vi "VI Tree.vi"   [LabVIEW 2014, in "KIT QV.lvlib"]
doc: "This is the instrument driver for the <INSTRUMENT NAME>. The VI Tree displays all the user-callable VIs of the instrument driver in an organized table."
uses:
  KIT QV.lvlib
panel:
  # "(c) 2015 GSI Helmholtzzentrum für Schwerionenforschung GmbH.  ALL RIGHTS RESERVED."
  # "SEE DIAGRAM\nFOR VI TREE."
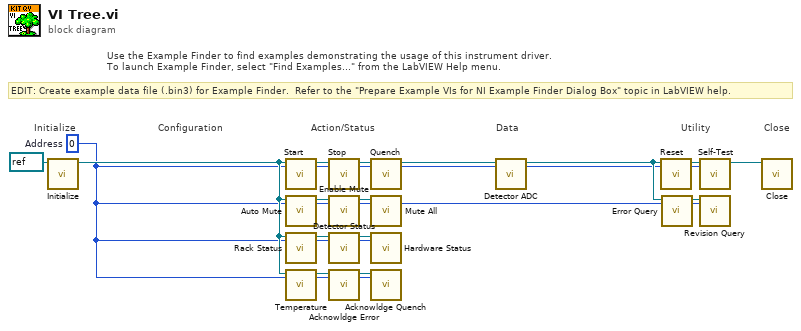
[diagram p0: block diagram]
diagram:
  w1 = u16 0  # Address
  # "EDIT: Create example data file (.bin3) for Example Finder.  Refer to the \"Prepare Example VIs for NI Example Finder Dialog Box\" topic in LabVIEW help."
  # "Use the Example Finder to find examples demonstrating the usage of this instrument driver.\nTo launch Example Finder, select \"Find Examples...\" from the LabVIEW Help menu."
  # "Configuration"
  # "Utility"
  # "Data"
  # "Action/Status"
  # "Close"
  # "Initialize"
  n1 = call "Initialize.vi"("VISA Resource Name"=refnum<visa-resource-name> refnum ("VISA resource name")) -> ("VISA Resource out"=w6:refnum<visa-resource-name>)  [unwired: 9 in, 1 out]
  n2 = call "Start.vi"("Address"=w1, "VISA Resource in"=w6) -> ("VISA Resource out"=w11:refnum<visa-resource-name>)  [unwired: 8 in, 1 out]
  n3 = call "Auto Mute.vi"("Address"=w1, "VISA Resource in"=w6) -> ("VISA Resource out"=w10:refnum<visa-resource-name>)  [unwired: 8 in, 1 out]
  n4 = call "Rack Status.vi"("Address"=w1, "VISA Resource in"=w6) -> ("VISA Resource out"=w8:refnum<visa-resource-name>)  [unwired: 6 in, 3 out]
  n5 = call "Temperature.vi"("Address"=w1, "VISA Resource in"=w6) -> ("VISA Resource out"=w3:refnum<visa-resource-name>)  [unwired: 7 in, 2 out]
  n6 = call "Stop.vi"("Address"=w1, "VISA Resource in"=w11) -> ("VISA Resource out"=w12:refnum<visa-resource-name>)  [unwired: 8 in, 1 out]
  n7 = call "Enable Mute.vi"("Address"=w1, "VISA Resource in"=w10) -> ("VISA Resource out"=w9:refnum<visa-resource-name>)  [unwired: 8 in, 1 out]
  n8 = call "Detector Status.vi"("Address"=w1, "VISA Resource in"=w8) -> ("VISA Resource out"=w7:refnum<visa-resource-name>)  [unwired: 6 in, 3 out]
  n9 = call "Acknowldge Error.vi"("Address"=w1, "VISA Resource in"=w3) -> ("VISA Resource out"=w2:refnum<visa-resource-name>)  [unwired: 8 in, 1 out]
  n10 = call "Quench.vi"("Address"=w1, "VISA Resource in"=w12) -> ("VISA Resource out"=w5:refnum<visa-resource-name>)  [unwired: 8 in, 1 out]
  n11 = call "Mute All.vi"("Address"=w1, "VISA Resource in"=w9) -> ()  [unwired: 8 in, 2 out]
  n12 = call "Hardware Status.vi"("Address"=w1, "VISA Resource in"=w7) -> ()  [unwired: 6 in, 4 out]
  n13 = call "Acknowldge Quench.vi"("Address"=w1, "VISA Resource in"=w2) -> ()  [unwired: 8 in, 2 out]
  n14 = call "Detector ADC.vi"("Address"=w1, "VISA Resource in"=w5) -> ("VISA Resource out"=w4:refnum<visa-resource-name>)  [unwired: 6 in, 3 out]
  n15 = call "Reset.vi"("Address"=w1, "VISA Resource in"=w4) -> ("VISA Resource out"=w15:refnum<visa-resource-name>)  [unwired: 8 in, 1 out]
  n16 = call "Error Query.vi"("Address"=w1, "VISA Resource in"=w4) -> ("VISA Resource in"=w13:refnum<visa-resource-name>)  [unwired: 6 in, 3 out]
  n17 = call "Self-Test.vi"("Address"=w1, "VISA Resource in"=w15) -> ("VISA Resource out"=w14:refnum<visa-resource-name>)  [unwired: 6 in, 3 out]
  n18 = call "Revision Query.vi"("Address"=w1, "VISA Resource in"=w13) -> ()  [unwired: 6 in, 4 out]
  n19 = call "Close.vi"("VISA Resource in"=w14) -> ()  [unwired: 10 in, 1 out]
